vi "Create.vi"(8 "error in (no error)":errorcluster, 10 "Action":T1=enum."Wait") -> (0 "error out":errorcluster, 3 "Action out":refnum<class "Action.lvclass">)   [LabVIEW 2013, in "PowderDeposition.lvlib" / "Action.lvclass"]
uses:
  Action.lvclass
  Motor-actions.ctl
  Wait/Wait.lvclass
  Main/Custom-errors.ctl
  Move-Timer/Move-Timer.lvclass
  Home/Home.lvclass
  Substrate/Substrate.lvclass
  Sieve/Sieve.lvclass
  Move-Absolute/Move-Absolute.lvclass
  Move-Relative/Move-Relative.lvclass
  Main/PD-Main.lvclass
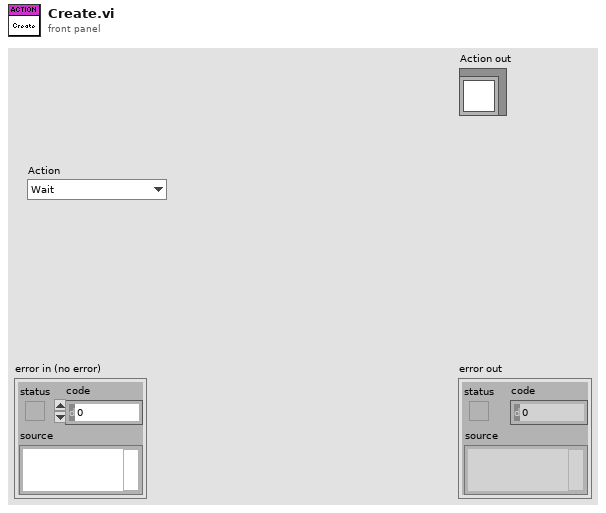
[diagram p1: front panel]
types:
  T1 = typedef "PowderDeposition.lvlib/Action.lvclass/Motor-actions.ctl" = enum16{"Move - Absolute", "Move - Relative", "Move - Timer", "Wait", "Home", "Substrate", "Sieve", "Stop"}
  T2 = typedef "PowderDeposition.lvlib/PD-Main.lvclass/Custom-errors.ctl" = enum16{"Not implemented", "Command not recognized", "Invalid input", "Timeout", "Load file failed", "Action failed", "Action invalid", "Motor inactive", "Not in range", "Unsafe state"}
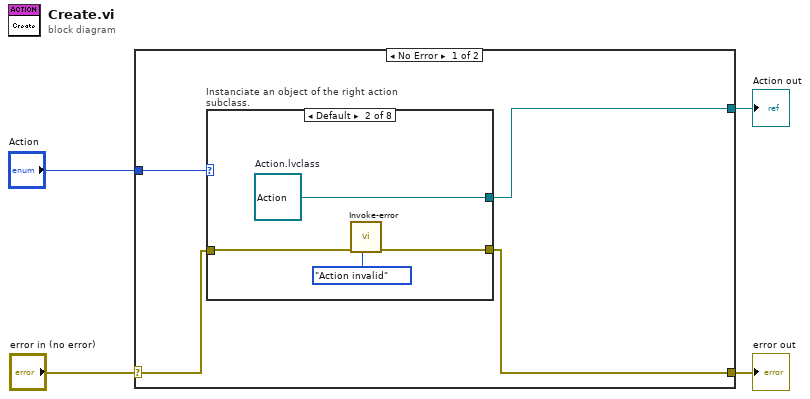
[diagram p0: block diagram]
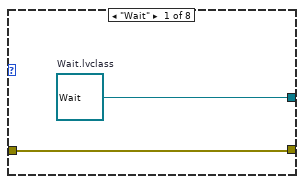
[diagram p2: hidden frame]
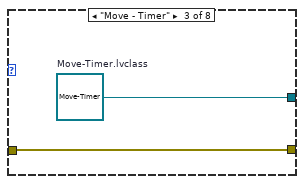
[diagram p3: hidden frame]
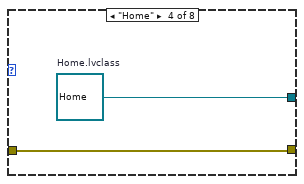
[diagram p4: hidden frame]
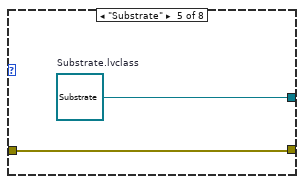
[diagram p5: hidden frame]
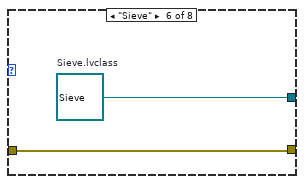
[diagram p6: hidden frame]
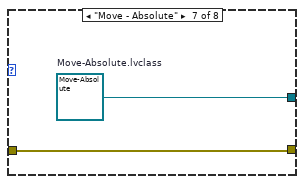
[diagram p7: hidden frame]
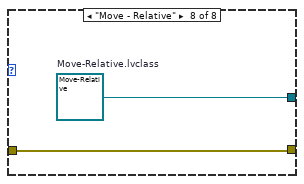
[diagram p8: hidden frame]
diagram:
  n1 = case shown="No Error" "error in (no error)" {
    selector: "error in (no error)" -> [w6 w27]
    tunnel: [w5 w27] -> w3
    tunnel: [w7 _] -> w2
    tunnel: "Action" -> [w8 _]
    frame No Error {
      n2 = case "Instanciate an object of the right action subclass." shown="Default" w8 {
        tunnel: [w10 w14 w16 w18 w20 w22 w24 w26] -> w7
        tunnel: w6 -> [w9 w12 w15 w17 w19 w21 w23 w25]
        tunnel: [w9 w11 w15 w17 w19 w21 w23 w25] -> w5
        frame "Wait" {
          w10 = refnum<class "Wait.lvclass"> refnum  # Wait.lvclass
        }
        frame Default {
          w14 = refnum<class "Action.lvclass"> refnum  # Action.lvclass
          n3 = call "Invoke-error.vi"("Error"=Custom-errors."Action invalid", "error in (no error)"=w12) -> ("error out"=w11:errorcluster)  [unwired: 9 in]
        }
        frame "Move - Timer" {
          w16 = refnum<class "Move-Timer.lvclass"> refnum  # Move-Timer.lvclass
        }
        frame "Home" {
          w18 = refnum<class "Home.lvclass"> refnum  # Home.lvclass
        }
        frame "Substrate" {
          w20 = refnum<class "Substrate.lvclass"> refnum  # Substrate.lvclass
        }
        frame "Sieve" {
          w22 = refnum<class "Sieve.lvclass"> refnum  # Sieve.lvclass
        }
        frame "Move - Absolute" {
          w24 = refnum<class "Move-Absolute.lvclass"> refnum  # Move-Absolute.lvclass
        }
        frame "Move - Relative" {
          w26 = refnum<class "Move-Relative.lvclass"> refnum  # Move-Relative.lvclass
        }
      }
    }
    frame Error {
    }
  }
  "error out" <- w3
  "Action out" <- w2
